vi "DisplacementRawConverterLoop.vi"   [LabVIEW 2016]
uses:
  <vilib>/rvi/Emulation/niFpgaGetClockAttributes.vi
  <vilib>/rvi/Emulation/niFpgaSctlEmulationGetInTimedLoop.vi
  <vilib>/rvi/Emulation/niFpgaEmulationReportErrorSimple.vi
  <vilib>/rvi/Emulation/niFpgaEmulationIsFPGAContextNoSignature.vi
  <vilib>/rvi/errors/niFpgaSetErrorForExecOnDevCompSimple.vi
  <vilib>/rvi/eio/common/nirviEmuReportErrorAndStop.vi
  <vilib>/rvi/DataTransferAndStorage/Container/Common/niFpgaContainerGetUniqueNameForEmu.vi
  <vilib>/rvi/FIFO/Fifo_Resource/nirvififoEmulationSetSize.vi
  <vilib>/rvi/FIFO/Fifo_Resource/nirviFifoEmulationQueueMgr.vi
  <instcachedir>/0/nirviFifoEmulationQueueMgr_E5CAEC123FF24DC58D834DCA3CDAA9B5.lvgen/nirviFifoEmulationQueueMgr_E5CAEC123FF24DC58D834DCA3CDAA9B5_028.vi
  <vilib>/Utility/error.llb/Clear Errors.vi
  <vilib>/rvi/FIFO/Fifo_Resource/nirvififoEmulationCreateLock.vi
  <vilib>/rvi/Emulation/niFpgaProcessEmulError.vi
  <vilib>/rvi/FIFO/Fifo_Resource/nirvififoEmulationObtainLock.vi
  <vilib>/rvi/FIFO/Fifo_Resource/nirvififoEmulationReleaseLock.vi
  <vilib>/rvi/occurrence/nirviWaitOnOccurrenceBase.vi
  <vilib>/rvi/errors/nirviReportUnexpectedCaseInternalError.vi
  <vilib>/rvi/errors/nirviReportUnexpectedCaseInternalError (U32).vi
  <userlib>/_NI FLP Library/FPGA/outsideSCTL/FlpLib Divide Shared Instance 0.vi
  <vilib>/rvi/FIFO/Fifo_Resource/nirvififoEmulationDetermineInputValidOut.vi
  <vilib>/rvi/Emulation/niFpgaCriticalErrorInLSC.vi
  <vilib>/rvi/DataTransferAndStorage/Container/XNode/niFpgaContainer.xnode
  <vilib>/rvi/FIFO/Fifo_Resource/nirvififoEmulationRead.vi
  <vilib>/rvi/FIFO/Fifo_Resource/nirvififoEmulationWrite.vi
types:
  T1 = cluster{"Timestamp":u64, "TxBytes":u64, "RxBytes":u64, "TxFrames":u64, "RxFrames":u64, "Sensor1Raw":i32, "Sensor2Raw":i32, "Sensor3Raw":i32, "Sensor4Raw":i32, "Sensor5Raw":i32, "Sensor6Raw":i32, "Sensor7Raw":i32, "Sensor8Raw":i32, "Sensor1Eng":sgl, "Sensor2Eng":sgl, "Sensor3Eng":sgl, "Sensor4Eng":sgl, "Sensor5Eng":sgl, "Sensor6Eng":sgl, "Sensor7Eng":sgl, "Sensor8Eng":sgl, "PositionX":sgl, "PositionY":sgl, "PositionZ":sgl, "RotationX":sgl, "RotationY":sgl, "RotationZ":sgl}
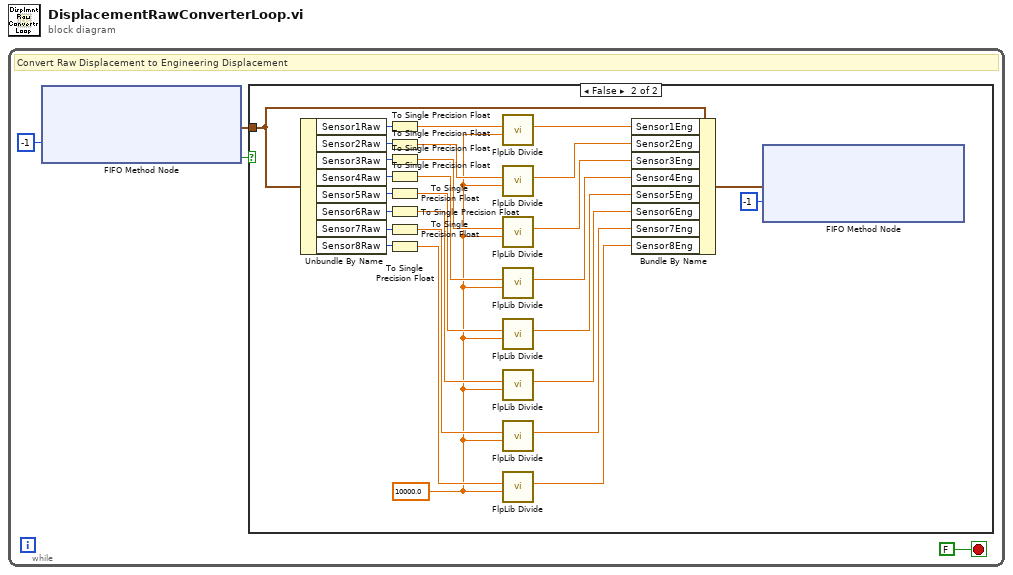
[diagram p0: block diagram]
diagram:
  n1 = while {
    stop <- FALSE stop-if-true
    # "Convert Raw Displacement to Engineering Displacement"
    n2 = xnode ("FIFO Method Node")("Timeout"=-1) -> ("Element"=w1:T1, "Timed Out?"=w3:bool)  [unwired: 1 in, 1 out]
    n3 = case shown="False" w3 {
      tunnel: w1 -> [_ w31]
      frame True {
      }
      frame False {
        w14 = sgl 10000.0
        n4 = Unbundle By Name(w31) -> ("Sensor1Raw"=w30:i32, "Sensor2Raw"=w29:i32, "Sensor3Raw"=w27:i32, "Sensor4Raw"=w25:i32, "Sensor5Raw"=w26:i32, "Sensor6Raw"=w24:i32, "Sensor7Raw"=w23:i32, "Sensor8Raw"=w28:i32)
        n5 = To Single Precision Float(number=w30) -> (single precision float=w22:sgl)
        n6 = To Single Precision Float(number=w29) -> (single precision float=w21:sgl)
        n7 = To Single Precision Float(number=w27) -> (single precision float=w20:sgl)
        n8 = To Single Precision Float(number=w25) -> (single precision float=w19:sgl)
        n9 = To Single Precision Float(number=w26) -> (single precision float=w18:sgl)
        n10 = To Single Precision Float(number=w24) -> (single precision float=w17:sgl)
        n11 = To Single Precision Float(number=w23) -> (single precision float=w16:sgl)
        n12 = To Single Precision Float(number=w28) -> (single precision float=w15:sgl)
        n13 = call-poly <userlib>:"FlpLib Divide.vi"("y"=w14, "x"=w22) -> ("x/y"=w13:sgl)  [unwired: 5 in]
        n14 = call-poly <userlib>:"FlpLib Divide.vi"("y"=w14, "x"=w21) -> ("x/y"=w12:sgl)  [unwired: 5 in]
        n15 = call-poly <userlib>:"FlpLib Divide.vi"("y"=w14, "x"=w20) -> ("x/y"=w11:sgl)  [unwired: 5 in]
        n16 = call-poly <userlib>:"FlpLib Divide.vi"("y"=w14, "x"=w19) -> ("x/y"=w10:sgl)  [unwired: 5 in]
        n17 = call-poly <userlib>:"FlpLib Divide.vi"("y"=w14, "x"=w18) -> ("x/y"=w9:sgl)  [unwired: 5 in]
        n18 = call-poly <userlib>:"FlpLib Divide.vi"("y"=w14, "x"=w17) -> ("x/y"=w8:sgl)  [unwired: 5 in]
        n19 = call-poly <userlib>:"FlpLib Divide.vi"("y"=w14, "x"=w16) -> ("x/y"=w7:sgl)  [unwired: 5 in]
        n20 = call-poly <userlib>:"FlpLib Divide.vi"("y"=w14, "x"=w15) -> ("x/y"=w6:sgl)  [unwired: 5 in]
        n21 = Bundle By Name(cluster=w31, "Sensor1Eng"=w13, "Sensor2Eng"=w12, "Sensor3Eng"=w11, "Sensor4Eng"=w10, "Sensor5Eng"=w9, "Sensor6Eng"=w8, "Sensor7Eng"=w7, "Sensor8Eng"=w6) -> (w5:T1)
        n22 = xnode ("FIFO Method Node")("Element"=w5, "Timeout"=-1) -> ()  [unwired: 1 in, 2 out]
      }
    }
  }
